vi "Launch SquareBattle.vi"   [LabVIEW 2020]
uses:
  SB App/SB App/SB App.lvclass
  Squares/Template/SquareTeam/MyTeam/MyTeam.lvclass
  C:/dev/illuminatedg/sol-squarebattle/SquareBattle/Team/Team.lvclass
  C:/dev/illuminatedg/sol-squarebattle/Squares/Template/SquareTeam/MyTeam/MyTeam.lvclass
panel:
  # "Run this VI to launch the app and test the unbuilt version of your team."
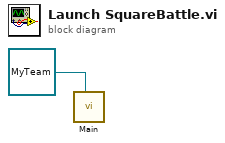
[diagram p0: block diagram]
diagram:
  n1 = call "Main.vi"("Dev Team"=refnum<class "MyTeam.lvclass"> refnum ("SquareTeam.lvlib:MyTeam.lvclass")) -> ()  [unwired: 11 in]
